vi "Reset Goal.vi"(8 "Error In":errorcluster, 10 "Time Goal (s)":dbl, 11 "Timer Handle":T1) -> (0 "Error Out":errorcluster, 3 "Timer Handle":T1)   [LabVIEW 2016, in "Timer Session.lvclass"]
doc: "Resets the timer. Allows to specify new time goal.\n\nYou can specify the input as timer name or timer reference. Using reference executes faster."
uses:
  Timer Session.lvclass
  Typedefs/Session Handle.ctl
  Timer Session.lvclass/Timer Session.ctl
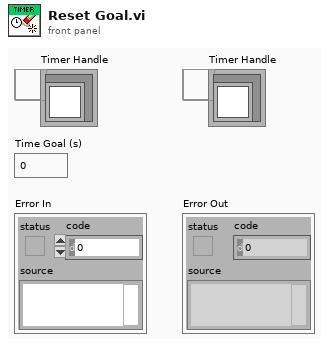
[diagram p1: front panel]
types:
  T1 = typedef "Timer Session.lvclass/Session Handle.ctl" = refnum<data-value>
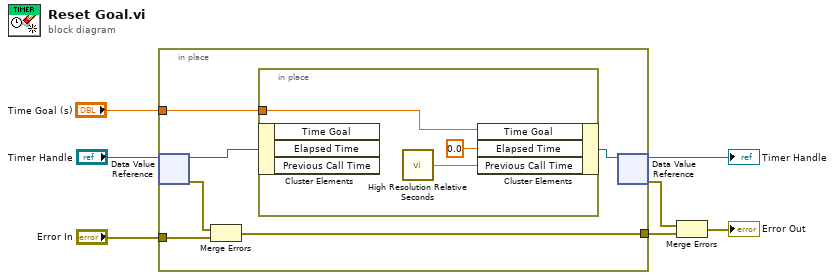
[diagram p0: block diagram]
diagram:
  n1 = in-place {
    in-place-border: "Error In" -> [w10]
    in-place-border: [w9] -> w5
    in-place-border: "Time Goal (s)" -> [w8]
    n2 = in-place-dvr #1("Timer Handle") -> (w13:refnum<class "Timer Session.lvclass">, w11:errorcluster)
    n3 = Merge Errors(w11, w10) -> (w9:errorcluster)
    n4 = in-place {
      in-place-border: w8 -> [w14]
      n5 = in-place-cluster #2(w13) -> ()  [unwired: 3 out]
      n6 = call <vilib>:"High Resolution Relative Seconds.vi"() -> ("relative seconds"=w15:dbl)
      n7 = in-place-cluster #2("Time Goal"=w14, "Elapsed Time"=0.0 ("Elapsed Time (s)"), "Previous Call Time"=w15) -> (w12:refnum<class "Timer Session.lvclass">)
    }
    n8 = in-place-dvr #1(w12) -> (→"Timer Handle":T1, w4:errorcluster)
  }
  n9 = Merge Errors(w4, w5) -> (→"Error Out":errorcluster)
